vi "Check_Sensor_Flame.vi"(8 "error in (no error)":errorcluster, 9 "NewVal":dbl, 10 "Data in":T1, 11 "Cluster in":refnum<vi>) -> (0 "error out":errorcluster, 2 "State":T2, 3 "Data out":T1)   [LabVIEW 2023]
uses:
  Controls/DataCluster.ctl
  Controls/State.ctl
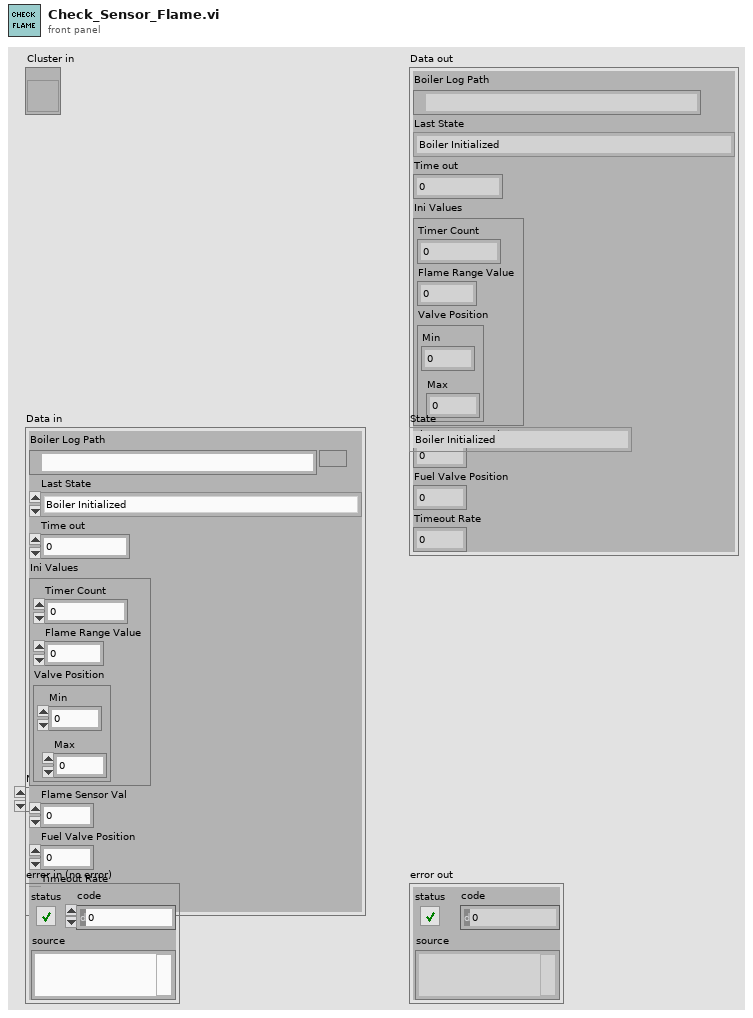
[diagram p1: front panel]
types:
  T1 = typedef "DataCluster.ctl" = cluster{"Boiler Log Path":path, "Last State":T2, "Time out":i32, "Ini Values":cluster{"Timer Count":dbl, "Flame Range Value":dbl, "Valve Position ":cluster{"Min":dbl, "Max":dbl}}, "Flame Sensor Val":dbl, "Fuel Valve Position":dbl, "Timeout Rate":i32}
  T2 = typedef "State.ctl" = enum16{"Boiler Initialized", "Boiler Ready", "Start Pre-Purge", "Pre-Purge Complete", "Pilot On", "Pilot Proved", "Force Draft Fan ON", "Boiler Running", "Start Shutdown Purge", "Shutdown Purge Complete", "Wait for Something"}
  T3 = typedef "Boiler Status Indicators.ctl" = cluster{"Status":string, "Primary Fan":bool, "Natural Gas Valve":bool, "Pilot":bool, "Fuel Valve":bool, "Forced Draft Fan":bool, "Time Count":dbl}
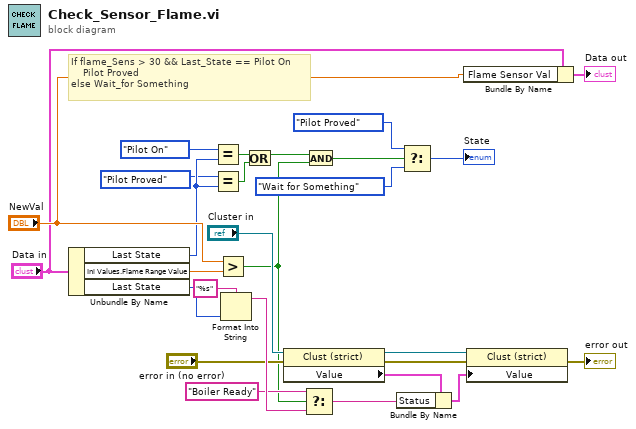
[diagram p0: block diagram]
diagram:
  # "If flame_Sens > 30 && Last_State == Pilot On\n    Pilot Proved\nelse Wait_for Something"
  n1 = Unbundle By Name("Data in") -> ("Last State"=w3:T2, "Ini Values.Flame Range Value"=w12:dbl, "Last State"=w23:T2)
  n2 = Equal?(x=State."Pilot On", y=w3) -> (x = y?=w6:bool)
  n3 = Equal?(x=State."Pilot Proved", y=w3) -> (x = y?=w1:bool)
  n4 = Greater?(x="NewVal", y=w12) -> (0:w8:bool)
  n5 = Format Into String(format string="%s", w23) -> (resulting string=w24:string)  [unwired: 2 in, 1 out]
  n6 = Or(x=w6, y=w1) -> (x .or. y?=w4:bool)
  n7 = property class="Clust (strict)"(reference="Cluster in", error in="error in (no error)") -> (reference out=w16:refnum<vi>, error out=w15:errorcluster, "Value"=w17:T3)
  n8 = Select(t="Boiler Ready", s=w8, f=w24) -> (s? t:f=w21:string)
  n9 = And(x=w4, y=w8) -> (x .and. y?=w9:bool)
  n10 = Bundle By Name(cluster=w17, "Status"=w21) -> (w18:T3)
  n11 = Select(t=State."Pilot Proved", s=w9, f=State."Wait for Something") -> (s? t:f=→"State":T2)
  n12 = Bundle By Name(cluster="Data in", "Flame Sensor Val"="NewVal") -> (→"Data out":T1)
  n13 = property class="Clust (strict)"(reference=w16, error in=w15, "Value"=w18) -> (error out=→"error out":errorcluster)  [unwired: 1 out]
